vi "Read buffer.vi"(8 "error in (no error)":errorcluster, 10 "pre-read delay(ms)":i16=-1, 11 "Serial Base in":refnum<class "Serial Base.lvclass">) -> (0 "error out":errorcluster, 1 "return count":u32, 2 "buffer output":string, 3 "Serial Base out":refnum<class "Serial Base.lvclass">)   [LabVIEW 2014, in "Serial Base.lvclass"]
doc: "<b>Description</b>\nReads the whole serial buffer from the device and returns the data in <b>buffer output</b>.\n\n------------------------------------------------------------------\n<b>pre-read delay(ms)</b>: miliseconds to wait, type <b>-1</b> to not wait\n<b>buffer output</b>: data returned in the buffer\n<b>bytes count</b>: contains the number of bytes actually read."
uses:
  Serial Base.lvclass
  Serial Base.lvclass/Serial Base.ctl
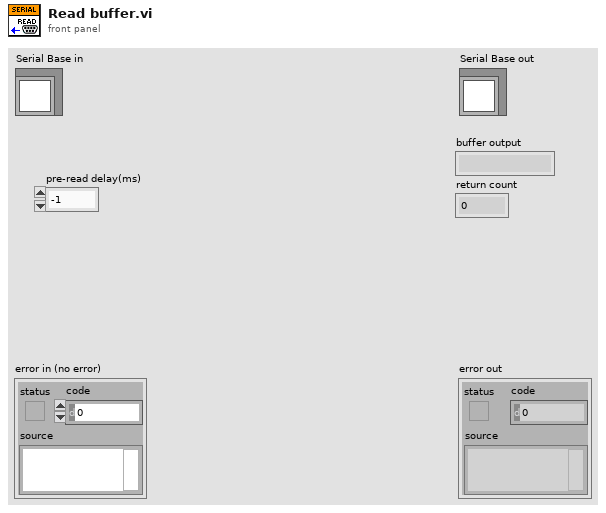
[diagram p1: front panel]
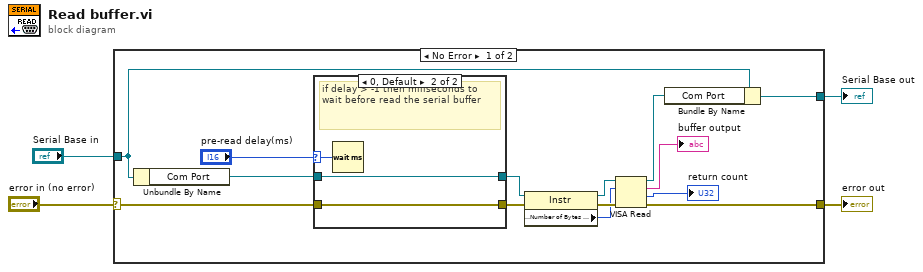
[diagram p0: block diagram]
diagram:
  n1 = case shown="No Error" "error in (no error)" {
    selector: "error in (no error)" -> [w6 w25]
    tunnel: [w10 w25] -> w3
    tunnel: [w17 w24] -> w1
    tunnel: "Serial Base in" -> [w18 w24]
    frame No Error {
      n2 = Unbundle By Name(w18) -> ("Com Port"=w8:refnum<visa-resource-name>)
      n3 = case shown="0, Default" "pre-read delay(ms)" {
        selector: "pre-read delay(ms)" -> [_ w21]
        tunnel: [w20 w23] -> w9
        tunnel: w8 -> [w20 w23]
        tunnel: w6 -> [w19 w22]
        tunnel: [w19 w22] -> w7
        frame -1 {
          # "-1 = not delay"
        }
        frame 0, Default {
          # "if delay > -1 then miliseconds to wait before read the serial buffer"
          n4 = Wait (ms)(milliseconds to wait=w21) -> ()  [unwired: 1 out]
        }
      }
      n5 = property class="Instr"(reference=w9, error in=w7) -> (reference out=w13:refnum<visa-resource-name>, error out=w12:errorcluster, "Serial Settings:Number of Bytes at Serial Port"=w11:u32)
      n6 = VISA Read(VISA resource name=w13, byte count=w11, error in (no error)=w12) -> (VISA resource name out=w14:refnum<visa-resource-name>, read buffer=→"buffer output":string, return count=→"return count":u32, error out=w10:errorcluster)
      n7 = Bundle By Name(cluster=w18, "Com Port"=w14) -> (w17:refnum<class "Serial Base.lvclass">)
    }
    frame Error {
    }
  }
  "error out" <- w3
  "Serial Base out" <- w1
